vi "Sonicator Tags.vi"(11 "SC Module Configs":T2[](array[typedef])) -> (2 "Sonicator Module Tags Array":T1[](array[typedef]), 3 "All Boolean Tags":string[](array[string]), 4 "All  Numeric Tags":string[](array[string]))   [LabVIEW 2018]
uses:
  Sonicator Module Folder/Feed Module/Controls/Sonicator Module Tag Names.ctl
  Sonicator Module Folder/Feed Module/Controls/Sonicator Module Config Cluster.ctl
  <vilib>/Utility/miscctls.llb/LVPoint32TypeDef.ctl
  Sonicator Module Folder/Feed Module/Controls/Sonicator Module Settings Cluster.ctl
  Sonic Systems P100/Sonic Systems P100 Settings.ctl
  Sonicator Module Folder/Sonicator Module.lvlib
  Sonic Systems P100/Sonic Systems P100.lvlib
panel:
  out "output cluster":T1
  # "Sonicator Settings"
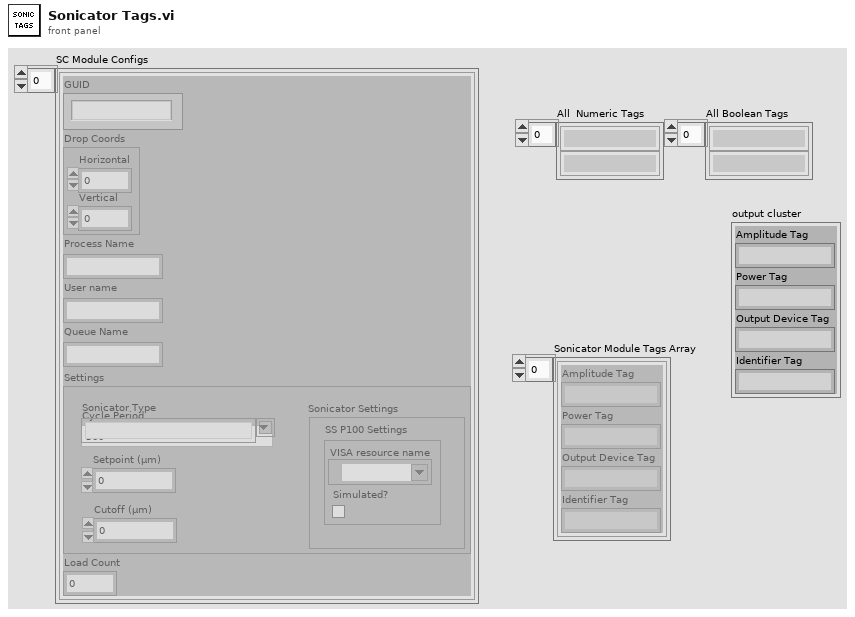
[diagram p1: front panel]
types:
  T1 = typedef "Sonicator Module.lvlib/Sonicator Module Tag Names.ctl" = cluster{"Amplitude Tag":string, "Power Tag":string, "Output Device Tag":string, "Identifier Tag":string}
  T2 = typedef "Sonicator Module.lvlib/Sonicator Module Config Cluster.ctl" = cluster{"GUID":string, "Drop Coords":T3, "Process Name":string, "User name":string, "Queue Name":string, "Settings":T4, "Load Count":i32}
  T3 = typedef "LVPoint32TypeDef.ctl" = cluster{"Horizontal":i32, "Vertical":i32}
  T4 = typedef "Sonicator Module.lvlib/Sonicator Module Settings Cluster.ctl" = cluster{"Cycle Period":dbl, "Sonicator Type":string, "SS P100 Settings":T5, "Setpoint (µm)":dbl, "Cutoff (W)":dbl}
  T5 = typedef "Sonic Systems P100.lvlib/Sonic Systems P100 Settings.ctl" = cluster{"VISA resource name":refnum<visa-resource-name>, "Simulated?":bool}
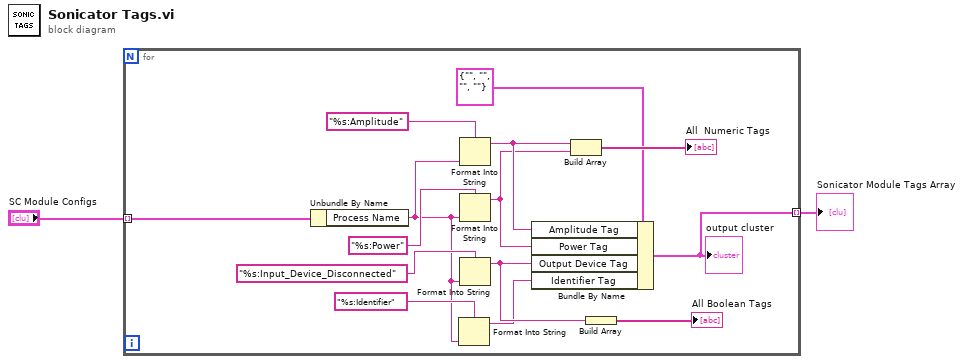
[diagram p0: block diagram]
diagram:
  n1 = for {
    tunnel: [w4] -> w2 mode=indexing
    tunnel: "SC Module Configs" -> [w8] mode=indexing
    n2 = Unbundle By Name(w8) -> ("Process Name"=w5:string)
    n3 = Format Into String(format string="%s:Identifier", w5) -> (resulting string=w3:string)  [unwired: 2 in, 1 out]
    n4 = Format Into String(format string="%s:Amplitude", w5) -> (resulting string=w13:string)  [unwired: 2 in, 1 out]
    n5 = Format Into String(format string="%s:Power", w5) -> (resulting string=w9:string)  [unwired: 2 in, 1 out]
    n6 = Format Into String(format string="%s:Input_Device_Disconnected", w5) -> (resulting string=w11:string)  [unwired: 2 in, 1 out]
    n7 = Bundle By Name(cluster=T1 {"Amplitude Tag"="", "Power Tag"="", "Output Device Tag"="", "Identifier Tag"=""} ("SC Tags"), "Amplitude Tag"=w13, "Power Tag"=w9, "Output Device Tag"=w11, "Identifier Tag"=w3) -> (w4:T1)
    "output cluster" <- w4
    n8 = Build Array(w13, w9) -> (→"All  Numeric Tags":string[])
    n9 = Build Array(w11) -> (→"All Boolean Tags":string[])
  }
  "Sonicator Module Tags Array" <- w2
